vi "Workshop Exercise 4 Solution.vi"() -> ()   [LabVIEW 2019]
doc: "This VI demonstrates how to programmatically change the state of the front panel window. \n\nThere are six states that are related to the front panel of a VI; Standard, Maximize, Minimize, Hidden, Closed and Invalid. All states are read/write with the exception of Invalid, which is read only. The Standard state sets the VI to its default front panel state. The Maximize state will maximize the VI to full screen size. Minimize state is used to minimize the VI to the task bar. When using the Hidden state, the VI is still in memory, yet the front panel is hidden from view. The Closed state will also hide the front panel of the VI, but the front panel objects of the VI are no longer in memory. Lastly, the Invalid state is returned if an attempt is made to apply a window state at a time when it cannot be applied to the VI."
uses:
  <vilib>/Utility/miscctls.llb/LVRectTypeDef.ctl
panel:
  out "Device Temperature":dbl=35.02
  out "Voltage Alarm Level Exceeded?":bool=TRUE
  in  "Stop":bool
  # "You can place in here any additional controls and indicators needed for debugging"
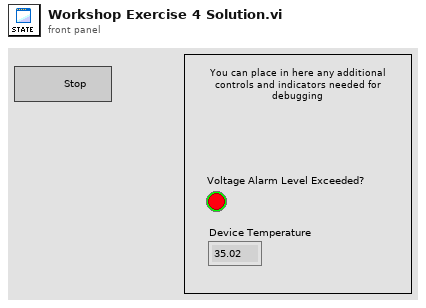
[diagram p1: front panel]
types:
  T1 = typedef "LVRectTypeDef.ctl" = cluster{"Left":i16, "Top":i16, "Right":i16, "Bottom":i16}
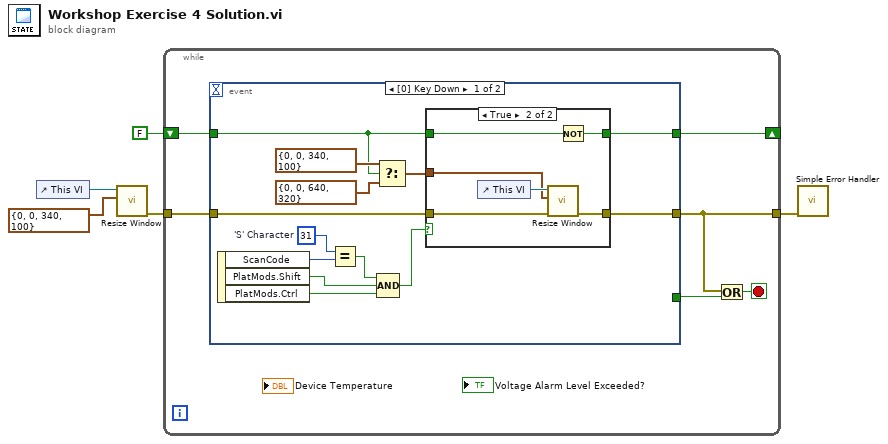
[diagram p0: block diagram]
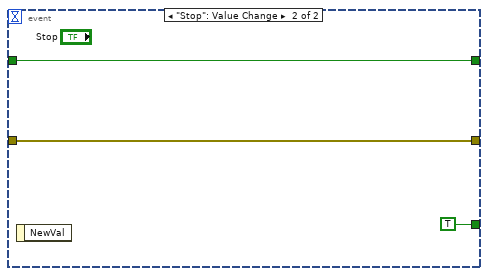
[diagram p3: hidden frame]
diagram:
  n1 = control-ref of="This VI"() -> (w3:refnum<vi>)
  n2 = call "Resize Window.vi"("Front Panel Window:Panel Bounds"=T1 {"Left"=0, "Top"=0, "Right"=340, "Bottom"=100}, "VI reference in"=w3) -> ("Error out"=w1:errorcluster)  [unwired: 8 in, 1 out]
  n3 = while {
    tunnel: [w9] -> w5
    tunnel: w1 -> [w8]
    shift-right: [w6] -> _
    shift-left: FALSE -> [w7]
    stop <- w10 stop-if-true
    # "Monitor User Interface Events"
    n4 = event shown="[0] Key Down" {
      selector: _ -> [_ _]
      dyn-events: _ -> [_ _]
      timeout: _ -> [_ _]
      tunnel: [_ TRUE ("T button?")] -> w11
      tunnel: [w17 w34] -> w9
      tunnel: w8 -> [w18 w34]
      tunnel: w7 -> [w13 w33]
      tunnel: [w16 w33] -> w6
      event Key Down {
        w24 = i16 31  # 'S' Character
        n5 = event-data() -> ("ScanCode"=w20:i16, "PlatMods.Shift"=w21:bool, "PlatMods.Ctrl"=w22:bool)  [unwired: 1 out]
        n6 = Equal?(x=w24, y=w20) -> (x = y?=w23:bool)
        n7 = Select(t=T1 {"Left"=0, "Top"=0, "Right"=340, "Bottom"=100} ("Front Panel Window:Panel Bounds"), s=w13, f=T1 {"Left"=0, "Top"=0, "Right"=640, "Bottom"=320} ("Front Panel Window:Panel Bounds")) -> (s? t:f=w12:T1)
        n8 = Compound Arithmetic op=AND(w23, w21, w22) -> (w19:bool)
        n9 = case shown="True" w19 {
          tunnel: w18 -> [w26 w31]
          tunnel: [w26 w30] -> w17
          tunnel: [w25 w28] -> w16
          tunnel: w13 -> [w25 w29]
          tunnel: w12 -> [_ w27]
          frame False {
          }
          frame True {
            n10 = control-ref of="This VI"() -> (w32:refnum<vi>)
            n11 = call "Resize Window.vi"("Error in"=w31, "Front Panel Window:Panel Bounds"=w27, "VI reference in"=w32) -> ("Error out"=w30:errorcluster)  [unwired: 7 in, 1 out]
            n12 = Not(x=w29) -> (.not. x?=w28:bool)
          }
        }
      }
      event "Stop": Value Change {
        # "Stop the VI."
        n13 = event-data() -> ()  [unwired: 2 out]
      }
    }
    n14 = Or(x=w9, y=w11) -> (x .or. y?=w10:bool)
  }
  n15 = call <vilib>:"Simple Error Handler.vi"("error in (no error)"=w5) -> ()  [unwired: 1 in, 8 out]
